vi "observacao.vi"() -> ()   [LabVIEW 2018, in "Shared_160.lvlib"] (continued)
                n1094 = case shown="True" w1420 {
                  selector: w1420 -> [_ w1423]
                  frame False {
                  }
                  frame True {
                    n1095 = Not(x=w1423) -> (.not. x?=w1422:bool)
                    n1096 = property on="Mensage Alarme" class="Str"("Visible"=FALSE) -> ()  [unwired: 2 in, 2 out]
                    n1097 = local write "Flag Alarm"(w1422) -> ()
                  }
                }
              }
            }
          }
          frame #13 {
            w1438 = u16 3 items=["Alarme", "Atencao", "Erro", "Ocupado", "Protecao", "Embreagem", "Tracking", "Var. Track", "Rápido", "Ligeiro", "Médio", "Lento", "Em movimento", ""] ("NomeStatus")
            w1439 = u16 3 items=["Alarme", "Atencao", "Erro", "Ocupado", "Protecao", "Embreagem", "Tracking", "Var. Track", "Rápido", "Ligeiro", "Médio", "Lento", "Em movimento", ""] ("NomeStatus")
            # "PROCESSO AQUISIÇÃO"
            n1098 = global read "Global_Telescopio.vi" "Correção Aquis"() -> (w1434:bool)
            n1099 = call "Bit Status AH.vi"("NomeStatus"=w1439) -> ("StatBit"=w1436:bool)
            n1100 = call "Bit Status DEC.vi"("NomeStatus"=w1438) -> ("StatBit"=w1437:bool)
            n1101 = Not Or(1:w1437, 2:w1436) -> (0:w1435:bool)
            n1102 = Compound Arithmetic op=AND(w1434, w1435) -> (w1440:bool)
            n1103 = case shown="True" w1440 {
              frame False {
              }
              frame True {
                # "Reseta Flag do movimento de\n offset do Sist de Aquisição"
                n1104 = global read "Global_Telescopio.vi" "CorrecaoMin"() -> (w1446:dbl)
                n1105 = global read "Global_Telescopio.vi" "aquis_asc"() -> (w1445:dbl)
                n1106 = global read "Global_Telescopio.vi" "aquis_dec"() -> (w1448:dbl)
                n1107 = Absolute Value(x=w1448) -> (abs(x)=w1444:dbl)
                n1108 = global read "Global_Telescopio.vi" "CorrecaoMin"() -> (w1449:dbl)
                n1109 = global write "Global_Telescopio.vi" "Correção Aquis"(FALSE ("Correção Aquis")) -> ()
                n1110 = Absolute Value(x=w1445) -> (abs(x)=w1443:dbl)
                n1111 = Greater?(x=w1444, y=w1449) -> (0:w1450:bool)
                n1112 = Greater?(x=w1443, y=w1446) -> (0:w1447:bool)
                n1113 = case shown="True" w1447 {
                  tunnel: w1445 -> [_ w1451]
                  frame False {
                  }
                  frame True {
                    w1453 = u16 1 items=["ZERO", "AH", "DEC", "TUBO", "CUP"] ("Controlador")
                    # "PROCESSO MOVE TELESCÓPIO"
                    n1114 = call "Conversao Ms to Hora texto.vi"("TRUE=HORA\nFALSE=GRAU"=TRUE ("TRUE=HORA\nFALSE=GRAU"), "PrecDEC"=w1451) -> ("Hora/Graus Texto Decimal"=w1456:string)
                    n1115 = call "Monta Comando.vi"("Set Point"=w1456, "Comando"="MOVER_REL", "Dispositivo"="EIXO" ("Comando"), "Controlador"=w1453) -> ()  [unwired: 1 in, 5 out]
                  }
                }
                n1116 = case shown="True" w1450 {
                  tunnel: w1448 -> [_ w1457]
                  frame False {
                  }
                  frame True {
                    w1459 = u16 2 items=["ZERO", "AH", "DEC", "TUBO", "CUP"] ("Controlador")
                    # "PROCESSO MOVE TELESCÓPIO"
                    n1117 = call "Conversao Ms to Hora texto.vi"("TRUE=HORA\nFALSE=GRAU"=FALSE ("TRUE=HORA\nFALSE=GRAU"), "PrecDEC"=w1457) -> ("Hora/Graus Texto Decimal"=w1462:string)
                    n1118 = call "Monta Comando.vi"("Set Point"=w1462, "Comando"="MOVER_REL", "Dispositivo"="EIXO" ("Comando"), "Controlador"=w1459) -> ()  [unwired: 1 in, 5 out]
                  }
                }
                n1119 = global write "Global_Telescopio.vi" "AQ Offset Mov"(TRUE ("AQ Offset Mov")) -> ()
              }
            }
          }
          frame #14 {
            w1475 = "\r\n"
            # "MUDANÇA 10/8/2010 \nIncluídos:\n- Nome do instrumento\n- RA do telescópio"
            # "OBS: O Arquivo é inicialmente apagado para \nEvitar que fique corrompido!"
            # "Escreve arquivo com Dados para o Uso da Página do PDA"
            n1120 = global read "Global_Telescopio.vi" "Lista Instrumentos"() -> (w1477:string[])
            n1121 = global read "Global_Telescopio.vi" "Sideral Time"() -> (w1467:dbl)
            n1122 = global read "Global_Telescopio.vi" "PosAH"() -> (w1468:dbl)
            n1123 = global read "Global_Telescopio.vi" "Instrum"() -> (w1476:u16)
            n1124 = local read "DOMO_ENC"() -> (w1489:string)
            n1125 = local read "CUP_STAT"() -> (w1485:string)
            n1126 = local read "AH_STAT"() -> (w1487:string)
            n1127 = local read "Sideral time"() -> (w1496:string)
            n1128 = local read "AH_ENC"() -> (w1491:string)
            n1129 = local read "UT"() -> (w1495:string)
            n1130 = Subtract(x=w1467, y=w1468) -> (x-y=w1472:dbl)
            n1131 = Add(x=6.283185307179586, y=w1472) -> (x+y=w1471:dbl)
            n1132 = Less Than 0?(x=w1472) -> (x < 0?=w1469:bool)
            n1133 = local read "TUBO_STAT"() -> (w1484:string)
            n1134 = call "Retira_tudo_depois_da_virgula.vi"("Entrada"=w1496) -> ("Saída"=w1493:string)
            n1135 = Format Date/Time String(time format string (%c)="%H:%M:%S") -> (date/time string=w1479:string)  [unwired: 2 in]
            n1136 = local read "FOCO_ENC"() -> (w1488:string)
            n1137 = local read "DEC_STAT"() -> (w1486:string)
            n1138 = local read "DEC_ENC"() -> (w1490:string)
            n1139 = Select(t=w1471, s=w1469, f=w1472) -> (s? t:f=w1473:dbl)
            n1140 = Index Array(array=w1477, index=w1476) -> (element=w1478:string)
            n1141 = Format Date/Time String(time format string (%c)="%d/%m/%Y") -> (date/time string=w1480:string)  [unwired: 2 in]
            n1142 = call "Retira_tudo_depois_da_virgula.vi"("Entrada"=w1495) -> ("Saída"=w1492:string)
            n1143 = call <vilib>:"Trim Whitespace.vi"("string"=w1493) -> ("trimmed string"=w1483:string)  [unwired: 1 in]
            n1144 = call "rad_hms.vi"("TRUE=HORA\nFALSE=GRAU"=TRUE, "Radiano"=w1473) -> ("Hora/Graus Texto Decimal"=w1466:string)  [unwired: 3 in]
            n1145 = String To Path(string="C:\\TCS\\ARQUIVOS\\DadosTCSPD.txt") -> (path=w1497:path)
            n1146 = Concatenate Strings(w1480, w1475, w1479, w1475, w1492, w1475, w1483, w1475, w1491, w1475, w1490, w1475, w1489, w1475, w1488, w1475, w1487, w1475, w1486, w1475, w1485, w1475, w1484, w1475, w1478, w1475, w1466, w1475) -> (w1499:string)
            n1147 = case shown="True" "Case Constant\n(See Context Help) 2" {
              tunnel: [w1508 w1511] -> w1498
              tunnel: w1497 -> [w1508 w1510]
              frame False {
              }
              frame True {
                n1148 = Delete(path (use dialog)=w1510) -> (deleted path=w1511:path, error out=→"error out":errorcluster)  [unwired: 4 in, 1 out]
              }
            }
            n1149 = call <vilib>:"Open_Create_Replace File.vi"("function (open:0)"=T8."open or create", "file path"=w1498) -> ("error out"=w1503:errorcluster, "refnum"=w1506:refnum<file>)  [unwired: 6 in, 2 out]
            n1150 = Set File Position(refnum=w1506, from (0:start)=enum16{"start", "end", "current"}."start" ("pos mode (0:2)"), error in=w1503) -> (refnum out=w1465:refnum<file>, error out=w1464:errorcluster)  [unwired: 1 in]
            n1151 = Write to Binary File(file (use dialog)=w1465, data=w1499, error in=w1464, 5:FALSE ("prepend array or string size? (T)")) -> (refnum out=w1505:refnum<file>, error out=w1504:errorcluster)  [unwired: 2 in, 1 out]
            n1152 = Close File(refnum=w1505, error in=w1504) -> (error out=w1507:errorcluster)  [unwired: 1 out]
            n1153 = call <vilib>:"Simple Error Handler.vi"("error in (no error)"=w1507) -> ()  [unwired: 4 in, 5 out]
          }
          frame #15 {
            # "Página do PDA"
            # "http://192.168.1.1:1080/pdaWeb/"
            # "TRATAMENTO DO PDA"
            n1154 = stacked-sequence {
              frame #0 {
                # "MUDANÇA  3/9/2010 \nIncluído case abaixo e código de seu estado TRUE para apagar eventuais comandos do PDA enviados antes do TCSPD rodar."
                n1155 = First Call?() -> (First Call?: T/F=w1512:bool)
                n1156 = case shown="True" w1512 {
                  frame False {
                    # "MUDANÇA  4/9/2010 \nSubstituída a VI \"New Read PPC\" pela \"Trata PDA\" a qual evita que o telescópio seja apontado para regiões proibidas (inclinação excessiva)."
                    # "lê e interpreta o arquivo ppc.txt"
                    n1157 = call "Trata PDA.vi"() -> ()  [unwired: 2 in]
                  }
                  frame True {
                    n1158 = call "Find ppctxt.vi"() -> ("Existe ppc.txt?"=w1514:bool, "ppc.txt Path"=w1513:path)  [unwired: 1 in]
                    n1159 = case shown="True" w1514 {
                      tunnel: w1513 -> [_ w1515]
                      frame False {
                      }
                      frame True {
                        # "limpa o arquivo ppc.txt"
                        n1160 = call "Wipe file.vi"("ppc path"=w1515) -> ()  [unwired: 2 out]
                      }
                    }
                  }
                }
              }
              frame #1 {
                n1161 = case shown="False" "Case Constant\n(See Context Help) 3" {
                  frame False {
                  }
                  frame True {
                    # "MUDANÇA:\nÉ necesário \nsubstituir as variáveis simuladas pelas do Sistema"
                    # "Simula os dados sendo alterados pela\nmovimentação do sistema"
                    n1162 = call "Data Table.vi"() -> ()  [unwired: 1 in]
                  }
                }
              }
              frame #2 {
                n1163 = case shown="True" "Case Constant\n(See Context Help) 4" {
                  frame False {
                  }
                  frame True {
                    # "Lê o arquivo padrão para o equip/o\nselecionado pelo PDA e grava o\narquivo ppcDisplay.htm adequado"
                    n1164 = call "Update Frame.vi"() -> ("Timeout"=w1518:u32)  [unwired: 2 in, 3 out]
                    n1165 = Wait Until Next ms Multiple(millisecond multiple=w1518) -> ()  [unwired: 1 out]
                  }
                }
              }
            }
          }
        }
        n1166 = global read "Global_Telescopio.vi" "Flag-Rotator"() -> (w99:bool)
        n1167 = case shown="True" w99 {
          frame False {
          }
          frame True {
            n1168 = local write "Setup, Pointing & Guiding"(T2."ROTATOR" ("Setup, Pointing & Guiding")) -> ()
          }
        }
      }
      frame #2 {
        n1169 = case shown="\"HANDSET\"" "Setup, Pointing & Guiding" {
          frame "POINTING", Default {
            n1170 = stacked-sequence {
              frame #0 {
                # "Clear Dados"
                n1171 = local read "ChkCalLocal"() -> (w1520:bool)
                n1172 = case shown="False" w1520 {
                  selector: w1520 -> [w1522 _]
                  frame False {
                    # "Para de Piscar/Blink\no botão"
                    n1173 = property on="ChkCalLocal" class="Bool (strict)"("Blinking"=w1522) -> ()  [unwired: 2 in, 2 out]
                  }
                  frame True {
                  }
                }
                n1174 = case shown="True" "BtPointObjClear" {
                  frame False {
                  }
                  frame True {
                    w1523 = ""
                    n1175 = local write "StrPointObjName"(w1523) -> ()
                    n1176 = local write "StrPointObjPMRA"(w1523) -> ()
                    n1177 = local write "StrPointObjPMDEC"(w1523) -> ()
                    n1178 = local write "StrPointObjRA"(w1523) -> ()
                    n1179 = local write "StrPointObjDEC"(w1523) -> ()
                    n1180 = local write "StrPointObjEpoch"(w1523) -> ()
                    n1181 = local write "StrPointTargetRA"(w1523) -> ()
                    n1182 = local write "StrPointTargetDEC"(w1523) -> ()
                  }
                }
              }
              frame #1 {
                # "20250910"
                # "20250910"
                # "A forma como os mostradores da janela TARGET são carregados está indefinida.\nVamos colocar um botão SET ao lado do botão CLEAR na janela OBJECT.\nQuando o botão SET for pressionado, os mostradores da janela TARGET\nseriam calculados a partir dos valores da janela OBJECT."
                n1183 = local read "StrPointObjRA"() -> (w1536:string)
                n1184 = local read "StrPointObjDEC"() -> (w1537:string)
                n1185 = local read "StrPointObjPMRA"() -> (w1527:string)
                n1186 = local read "StrPointObjPMDEC"() -> (w1526:string)
                n1187 = local read "Temp amb"() -> (w1542:string)
                n1188 = local read "pressão atm"() -> (w1541:string)
                n1189 = local read "hum local"() -> (w1540:string)
                n1190 = call "Check coord input.vi"("coordIn"=w1536, "RA=T, default: F=DEC"=TRUE) -> ("coordOut"=w1532:string, "valid"=w1531:bool)  [unwired: 8 in]
                n1191 = call "Check coord input.vi"("coordIn"=w1537, "RA=T, default: F=DEC"=FALSE) -> ("coordOut"=w1535:string, "valid"=w1534:bool)  [unwired: 8 in]
                n1192 = call "Arcsec to Rad_ String.vi"("VAR ARCSEC"=w1527) -> ("VAR RAD"=w1529:string, "valid"=w1524:bool)  [unwired: 5 in]
                n1193 = call "Arcsec to Rad_ String.vi"("VAR ARCSEC"=w1526) -> ("VAR RAD"=w1528:string, "valid"=w1525:bool)  [unwired: 5 in]
                n1194 = Compound Arithmetic op=AND("BtPointPrecess", w1531, w1534, w1524, w1525) -> (w1539:bool)
                n1195 = case shown="True" w1539 {
                  tunnel: w1532 -> [_ w1551]
                  tunnel: w1535 -> [_ w1550]
                  tunnel: w1542 -> [_ w1549]
                  tunnel: w1541 -> [_ w1548]
                  tunnel: w1540 -> [_ w1547]
                  tunnel: w1529 -> [_ w1546]
                  tunnel: w1528 -> [_ w1545]
                  tunnel: "BtPointPrecess" -> [w1543 _]
                  frame False {
                    n1196 = case shown="True" w1543 {
                      frame False {
                      }
                      frame True {
                        n1197 = One Button Dialog(message="Entrada inválida.\nInvalid data entry") -> ()  [unwired: 1 in, 1 out]
                      }
                    }
                  }
                  frame True {
                    n1198 = stacked-sequence {
                      tunnel: w1551 -> [w1587 _ _]
                      tunnel: w1550 -> [w1585 _ _]
                      tunnel: w1549 -> [w1595 _ _]
                      tunnel: w1548 -> [w1594 _ _]
                      tunnel: w1547 -> [w1593 _ _]
                      tunnel: w1546 -> [w1559 _ _]
                      tunnel: w1545 -> [w1558 _ _]
                      frame #0 {
                        # "PROCESSO PRECESSÃO"
                        # "MUDANÇA:\nVI Botao SET trocada por Botao Precess, eliminando entrada do Frame de coord. (Mean, Topo, Geo)"
                        n1199 = local read "ChkPointPrecessed"() -> (w1567:bool)
                        n1200 = call "Comma_to_Point.vi"("Lat_A"=w1585) -> ("Saída"=w1581:string)
                        n1201 = call "Comma_to_Point.vi"("Lat_A"=w1587) -> ("Saída"=w1583:string)
                        n1202 = call "hms_rad.vi"("True = hora"=FALSE, "Texto Graus"=w1581) -> ("radianos"=w1554:dbl)  [unwired: 3 in]
                        n1203 = call "hms_rad.vi"("True = hora"=TRUE, "Texto Graus"=w1583) -> ("radianos"=w1557:dbl)  [unwired: 3 in]
                        n1204 = call "rad_hms.vi"("TRUE=HORA\nFALSE=GRAU"=TRUE ("TRUE=HORA\nFALSE=GRAU"), "Radiano"=w1557) -> ("Hora/Graus Texto Decimal"=w1555:string)  [unwired: 3 in]
                        n1205 = call "rad_hms.vi"("TRUE=HORA\nFALSE=GRAU"=FALSE ("TRUE=HORA\nFALSE=GRAU"), "Radiano"=w1554) -> ("Hora/Graus Texto Decimal"=w1553:string)  [unwired: 3 in]
                        n1206 = call "Comma_to_Point.vi"("Lat_A"=w1594) -> ("Saída"=w1565:string)
                        n1207 = call "Comma_to_Point.vi"("Lat_A"=w1593) -> ("Saída"=w1564:string)
                        n1208 = call "Comma_to_Point.vi"("Lat_A"=w1595) -> ("Saída"=w1566:string)
                        n1209 = global write "Global_Telescopio.vi" "pubRaAcquis"(w1555) -> ()
                        n1210 = global write "Global_Telescopio.vi" "pubDecAcquis"(w1553) -> ()
                        n1211 = Number To Fractional String(use system decimal point (T)=FALSE, number=w1554, precision (6)=i16 9) -> (F-format string=w1570:string)  [unwired: 1 in]
                        n1212 = Number To Fractional String(use system decimal point (T)=FALSE, number=w1557, precision (6)=i16 9) -> (F-format string=w1571:string)  [unwired: 1 in]
                        n1213 = call "Botão Precess.vi"("AR"=w1571, "Precessed Coord."=w1567, "Dec"=w1570, "Temp local amb(K)"=w1566, "Pressao atm local (mB)"=w1565, "Hum rel local"=w1564, "Var RA"=w1559, "Var DEC"=w1558) -> ("RA"=w1597:dbl, "DEC"=w1560:dbl, "Hora Sideral (rad)"=w1596:dbl, "Dist. Zenital (rad)"=w1569:dbl, "Observed HA (radians)"=→"HA obs":dbl, "Massa de Ar"=w1568:dbl)  [unwired: 2 in]
                        "RA obs" <- w1597
                        "DEC obs" <- w1560
                        n1214 = local write "Zenital angle"(w1569) -> ()
                        n1215 = call "rad_hms.vi"("TRUE=HORA\nFALSE=GRAU"=FALSE ("TRUE=HORA\nFALSE=GRAU"), "Radiano"=w1560) -> ("Hora/Graus Texto Decimal"=w1577:string)  [unwired: 3 in]
                        n1216 = call "rad-graus.vi"("Radiano"=w1569) -> ("Graus"=w1592:dbl)
                        n1217 = Number To Fractional String(number=w1568, precision (6)=i16 3) -> (F-format string=→"Air Mass":string)  [unwired: 2 in]
                        n1218 = Number To Fractional String(number=w1592, precision (6)=i16 1) -> (F-format string=→"Zenital Angle":string)  [unwired: 2 in]
                        n1219 = call "rad_hms.vi"("TRUE=HORA\nFALSE=GRAU"=TRUE ("TRUE=HORA"), "Radiano"=w1597) -> ("Hora/Graus Texto Decimal"=w1579:string)  [unwired: 3 in]
                        n1220 = local write "StrPointTargetDEC"(w1577) -> ()
                        n1221 = local write "StrPointTargetRA"(w1579) -> ()
                        n1222 = disable-structure shown="Disabled" {
                          disable-tunnel: [w1601 _] -> _
                          disable-tunnel: w1597 -> [w1600 _]
                          disable-tunnel: w1596 -> [w1599 _]
                          disable-tunnel: w1560 -> [w1598 _]
                          frame Disabled {
                            n1223 = call "Hora_Limite.vi"("Asc Reta RA rad"=w1600, "Sideral Time rad"=w1599, "Declinação rad"=w1598) -> ("TO Tempo de Observação Horas"=w1601:dbl)  [unwired: 2 in]
                          }
                          frame Enabled {
                          }
                        }
                        n1224 = call "Novo_tempo_obs_inicial.vi"("TS"=w1596, "RA"=w1597, "DEC"=w1560) -> ("TO rad"=w1561:dbl)  [unwired: 7 in, 1 out]
                        n1225 = case shown="True" "TRUE=HORA\nFALSE=GRAU" {
                          frame False {
                          }
                          frame True {
                            # "Sincroniza hora do\nPC com GPS"
                            n1226 = call "About_Time.vi"() -> ()  [unwired: 1 in]
                          }
                        }
                        n1227 = call "rad_hms.vi"("TRUE=HORA\nFALSE=GRAU"=TRUE ("TRUE=HORA\nFALSE=GRAU"), "Radiano"=w1561) -> ("Hora/Graus Texto Decimal"=→"Tempo Obs":string)  [unwired: 3 in]
                      }
                      frame #1 {
                        # "Testa o ângulo zenital menor que 70º o led \"Working Area\" \naceso na cor verde se o ângulozenital menor que 70º e \nvermelho em caso cont rário."
                        n1228 = global read "Global_Telescopio.vi" "Piscar working area"() -> (w1608:bool)
                        n1229 = global read "Global_Telescopio.vi" "working area = VERDE"() -> (w1607:bool)
                        n1230 = global read "Global_Telescopio.vi" "ativar botão GO"() -> (w1605:bool)
                        n1231 = case shown="True" w1607 {
                          frame False {
                            # "False=Vermelho"
                            n1232 = local write "LedPointWorkArea"(FALSE ("LedPointWorkArea")) -> ()
                          }
                          frame True {
                            # "True=Verde"
                            "LedPointWorkArea" <- TRUE ("LedPointWorkArea")
                          }
                        }
                        n1233 = global write "Global_Telescopio.vi" "Botão GO = STOP"(FALSE ("Botão GO = STOP")) -> ()
                        n1234 = case shown="True" w1605 {
                          selector: w1605 -> [_ w1609]
                          frame False {
                          }
                          frame True {
                            n1235 = property on="BtTargetPoint" class="Bool"("Visible"=w1609) -> ()  [unwired: 2 in, 2 out]
                          }
                        }
                        n1236 = global write "Global_Telescopio.vi" "Piscar working area"(w1608) -> ()
                        n1237 = global read "Global_Telescopio.vi" "desativar botão GO"() -> (w1606:bool)
                        n1238 = case shown="True" w1606 {
                          selector: w1606 -> [_ w1611]
                          frame False {
                          }
                          frame True {
                            n1239 = Not(x=w1611) -> (.not. x?=w1610:bool)
                            n1240 = property on="BtTargetPoint" class="Bool"("Visible"=w1610) -> ()  [unwired: 2 in, 2 out]
                          }
                        }
                        n1241 = property on="LedPointWorkArea" class="Bool (strict)"("Visible"=TRUE ("Botão GO = STOP")) -> ()  [unwired: 2 in, 2 out]
                        n1242 = property on="LedPointing" class="Bool (strict)"("Visible"=FALSE) -> ()  [unwired: 2 in, 2 out]
                      }
                      frame #2 {
                        n1243 = global read "Global_Telescopio.vi" "CalDEC Local"() -> (w1619:dbl)
                        n1244 = global read "Global_Telescopio.vi" "CalAH Local"() -> (w1620:dbl)
                        n1245 = local read "ChkCalLocal"() -> (w1614:bool)
                        n1246 = Not Equal To 0?(x=w1620) -> (x != 0?=w1617:bool)
                        n1247 = Not Equal To 0?(x=w1619) -> (x != 0?=w1618:bool)
                        n1248 = Or(x=w1617, y=w1618) -> (x .or. y?=w1615:bool)
                        n1249 = And(x=w1614, y=w1615) -> (x .and. y?=w1616:bool)
                        n1250 = case shown="True" w1616 {
                          frame False {
                          }
                          frame True {
                            n1251 = local read "HA obs"() -> (w1640:dbl)
                            n1252 = local read "DEC obs"() -> (w1634:dbl)
                            n1253 = global read "Global_Telescopio.vi" "AH Zero Local"() -> (w1638:dbl)
                            n1254 = global read "Global_Telescopio.vi" "DEC Zero Local"() -> (w1633:dbl)
                            n1255 = global read "Global_Telescopio.vi" "Raio Máximo"() -> (w1622:dbl)
                            n1256 = Cosine(x=w1634) -> (cos(x)=w1639:dbl)
                            n1257 = Cosine(x=w1633) -> (cos(x)=w1637:dbl)
                            n1258 = Multiply(x=w1640, y=w1639) -> (x*y=w1636:dbl)
                            n1259 = Multiply(x=w1638, y=w1637) -> (x*y=w1635:dbl)
                            n1260 = Subtract(x=w1634, y=w1633) -> (x-y=w1629:dbl)
                            n1261 = Multiply(x=w1629, y=w1629) -> (x*y=w1632:dbl)
                            n1262 = Subtract(x=w1636, y=w1635) -> (x-y=w1628:dbl)
                            n1263 = Multiply(x=w1628, y=w1628) -> (x*y=w1630:dbl)
                            n1264 = Add(x=w1630, y=w1632) -> (x+y=w1631:dbl)
                            n1265 = Square Root(x=w1631) -> (sqrt(x)=w1627:dbl)
                            n1266 = Multiply(x=w1627, y=180.0) -> (x*y=w1625:dbl)
                            n1267 = Divide(x=w1625, y=3.141592653589793) -> (x/y=w1623:dbl)
                            n1268 = Greater?(x=w1623, y=w1622) -> (0:w1621:bool)
                            n1269 = property on="ChkCalLocal" class="Bool (strict)"("Blinking"=w1621) -> ()  [unwired: 2 in, 2 out]
                          }
                        }
                      }
                    }
                  }
                }
              }
              frame #2 {
                # "20250910"
                # "Clicando-se essa Tecla\nInicia-se o Apontamento"
                n1270 = local read "StrPointObjRA"() -> (w1655:string)
                n1271 = local read "StrPointObjDEC"() -> (w1652:string)
                n1272 = local read "StrPointObjPMRA"() -> (w1642:string)
                n1273 = local read "StrPointObjPMDEC"() -> (w1643:string)
                n1274 = local read "Temp amb"() -> (w1658:string)
                n1275 = local read "pressão atm"() -> (w1657:string)
                n1276 = local read "hum local"() -> (w1663:string)
                n1277 = control-ref of="BtTargetPoint"() -> (w1660:refnum<vi>)
                n1278 = property class="Bool"(reference=w1660) -> ("Boolean Text.Text"=w1661:string)  [unwired: 1 in, 2 out]
                n1279 = call "Check coord input.vi"("coordIn"=w1655, "RA=T, default: F=DEC"=TRUE) -> ("coordOut"=w1653:string, "valid"=w1649:bool)  [unwired: 8 in]
                n1280 = call "Check coord input.vi"("coordIn"=w1652, "RA=T, default: F=DEC"=FALSE) -> ("coordOut"=w1651:string, "valid"=w1648:bool)  [unwired: 8 in]
                n1281 = call "Arcsec to Rad_ String.vi"("VAR ARCSEC"=w1642) -> ("VAR RAD"=w1644:string, "valid"=w1646:bool)  [unwired: 5 in]
                n1282 = call "Arcsec to Rad_ String.vi"("VAR ARCSEC"=w1643) -> ("VAR RAD"=w1645:string, "valid"=w1647:bool)  [unwired: 5 in]
                n1283 = Equal?(x=w1661, y="POINT") -> (x = y?=w1659:bool)
                n1284 = Compound Arithmetic op=AND("BtTargetPoint", w1649, w1648, w1646, w1647) -> (w1656:bool)
                n1285 = case shown="True" w1656 {
                  tunnel: w1653 -> [_ w1670]
                  tunnel: w1651 -> [_ w1674]
                  tunnel: w1658 -> [_ w1671]
                  tunnel: w1657 -> [_ w1672]
                  tunnel: w1663 -> [_ w1673]
                  tunnel: w1659 -> [_ w1668]
                  tunnel: w1645 -> [_ w1667]
                  tunnel: w1644 -> [_ w1666]
                  tunnel: "BtTargetPoint" -> [w1664 _]
                  frame False {
                    n1286 = case shown="True" w1664 {
                      frame False {
                      }
                      frame True {
                        n1287 = One Button Dialog(message="Entrada inválida.\nInvalid data entry") -> ()  [unwired: 1 in, 1 out]
                      }
                    }
                  }
                  frame True {
                    n1288 = case shown="True" w1668 {
                      selector: w1668 -> [w1676 _]
                      tunnel: w1674 -> [_ w1700]
                      tunnel: w1673 -> [_ w1686]
                      tunnel: w1672 -> [_ w1685]
                      tunnel: w1671 -> [_ w1684]
                      tunnel: w1670 -> [_ w1699]
                      tunnel: w1667 -> [_ w1679]
                      tunnel: w1666 -> [_ w1680]
                      frame False {
                        w1677 = 0 ("estado")
                        # "Zera Máquina de Estado\nPelo Botão STOP"
                        n1289 = Not(x=w1676) -> (.not. x?=w1678:bool)
                        n1290 = local write "LedPointing"(w1676) -> ()
                        n1291 = global write "Global_Telescopio.vi" "Botão GO = STOP"(w1678) -> ()
                        n1292 = call "Stop.vi"() -> ()  [unwired: 1 in, 1 out]
                        n1293 = local write "statDEC"(w1677) -> ()
                        n1294 = local write "statAH"(w1677) -> ()
                        n1295 = local write "statCUP"(w1677) -> ()
                        "Flag Stop" <- TRUE ("Flag Stop")
                      }
                      frame True {
                        w1681 = ""
                        w1698 = FALSE ("use system decimal point (T)")
                        n1296 = call "Comma_to_Point.vi"("Lat_A"=w1699) -> ("Saída"=w1694:string)
                        n1297 = call "Comma_to_Point.vi"("Lat_A"=w1700) -> ("Saída"=w1695:string)
                        n1298 = call "hms_rad.vi"("True = hora"=TRUE, "Texto Graus"=w1694) -> ("radianos"=w1703:dbl)  [unwired: 3 in]
                        n1299 = call "hms_rad.vi"("True = hora"=FALSE, "Texto Graus"=w1695) -> ("radianos"=w1701:dbl)  [unwired: 3 in]
                        n1300 = local write "NAME"(w1681) -> ()
                        n1301 = local write "RA"(w1681) -> ()
                        n1302 = local write "DEC"(w1681) -> ()
                        n1303 = Number To Fractional String(use system decimal point (T)=w1698, number=w1703, precision (6)=i16 9) -> (F-format string=w1683:string)  [unwired: 1 in]
                        n1304 = Number To Fractional String(use system decimal point (T)=w1698, number=w1701, precision (6)=i16 9) -> (F-format string=w1682:string)  [unwired: 1 in]
                        n1305 = call "PrecessaoCorrigida.vi"("Coordenada do dia"="ChkPointPrecessed", "HabCorrModelo"="ChkModel", "UseLocalZero"="ChkCalLocal", "UseGlobalZero"="ChkCalGlobal", "RA"=w1683, "DEC"=w1682, "MovProprioRA"=w1680, "MovProprioDEC"=w1679, "Temp amb (K)"=w1684, "Press atm (mB)"=w1685, "Humid relat"=w1686) -> ("Estado"=w1689:i32, "RA"=w1688:dbl, "DEC"=w1687:dbl)  [unwired: 2 out]
                        n1306 = Equal To 0?(x=w1689) -> (x = 0?=w1696:bool)
                        n1307 = case shown="False" w1696 {
                          selector: w1696 -> [w1719 _]
                          tunnel: "ChkCalLocal" -> [w1731 _]
                          tunnel: "ChkCalGlobal" -> [w1730 _]
                          tunnel: w1682 -> [w1729 _]
                          tunnel: w1683 -> [w1728 _]
                          tunnel: w1679 -> [w1725 _]
                          tunnel: w1680 -> [w1724 _]
                          tunnel: w1689 -> [w1706 _]
                          tunnel: w1688 -> [w1727 _]
                          tunnel: w1687 -> [w1726 _]
                          tunnel: "ChkPointPrecessed" -> [w1722 _]
                          frame False {
                            w1709 = FALSE ("Coude")
                            w1710 = FALSE ("WeakSel")
                            w1711 = T5."Enabled" ("Disabled")
                            w1712 = TRUE ("MOUNT")
                            w1723 = 0 ("M_AH")
                            w1720 = TRUE
                            # "ABAS DE CONTROLE"
                            # "MUDANÇA:\nIncluído CASE"
                            # "Seta máquinas de\nestado aba ÚTILS"
                            n1308 = global write "Global_Telescopio.vi" "CoordDia"(w1722) -> ()
                            n1309 = global write "Global_Telescopio.vi" "CalGlobal"(w1730) -> ()
                            n1310 = global write "Global_Telescopio.vi" "CalLocal"(w1731) -> ()
                            n1311 = call "Envia LOG.vi"() -> ()  [unwired: 8 in, 2 out]
                            n1312 = global write "Global_Telescopio.vi" "TargetRA"(w1727) -> ()
                            n1313 = global write "Global_Telescopio.vi" "TargetDEC"(w1726) -> ()
                            n1314 = local write "statAH"(w1706) -> ()
                            n1315 = property on="LedPointWorkArea" class="Bool (strict)"("Visible"=FALSE ("Botão GO = STOP")) -> ()  [unwired: 2 in, 2 out]
                            n1316 = local write "statDEC"(w1706) -> ()
                            n1317 = global write "Global_Telescopio.vi" "ObjCentrado"(w1719) -> ()
                            n1318 = local write "RA on Target"(w1719) -> ()
                            n1319 = local write "DEC on Target"(w1719) -> ()
                            n1320 = local write "Dome on Target"(w1719) -> ()
                            n1321 = local read "ChkDomeEnable"() -> (w1718:bool)
                            n1322 = local write "M_AH"(w1723) -> ()
                            n1323 = local write "M_DEC"(w1723) -> ()
                            n1324 = local write "M_CUP"(w1723) -> ()
                            n1325 = case shown="True" w1718 {
                              selector: w1718 -> [w1752 _]
                              tunnel: w1706 -> [_ w1754]
                              tunnel: [0 ("Estado") w1754] -> w1717
                              tunnel: [u8 2 ("Disabled") u8 0 ("Disabled")] -> w1716
                              frame False {
                                n1326 = local write "DOME"(w1752) -> ()
                              }
                              frame True {
                              }
                            }
                            n1327 = Tick Count (ms)() -> (millisecond timer value=w1714:u32)
                            n1328 = Add(x=w1714, y=u32 120000) -> (x+y=w1715:u32)
                            n1329 = local write "Tick Cupula"(w1715) -> ()
                            n1330 = local write "MOUNT"(w1712) -> ()
                            n1331 = local write "GUIDER"(w1712) -> ()
                            n1332 = property on="LedPointing" class="Bool (strict)"("Visible"=w1720) -> ()  [unwired: 2 in, 2 out]
                            n1333 = local write "statCUP"(w1717) -> ()
                            n1334 = property on="DOME" class="Bool (strict)"("Disabled"=w1716) -> ()  [unwired: 2 in, 2 out]
                            n1335 = stacked-sequence {
                              frame #0 {
                                n1336 = local read "StrPointObjName"() -> (w1732:string)
                                n1337 = local read "StrPointObjRA"() -> (w1733:string)
                                n1338 = local read "StrPointObjDEC"() -> (w1734:string)
                                n1339 = global write "Global_Telescopio.vi" "NAME OBJETO AUX"(w1732) -> ()
                                n1340 = global write "Global_Telescopio.vi" "RA AUX"(w1733) -> ()
                                n1341 = global write "Global_Telescopio.vi" "DEC AUX"(w1734) -> ()
                              }
                              frame #1 {
                                w1736 = u16 4 items=["ZERO", "AH", "DEC", "TUBO", "CUP"] ("Controlador")
                                n1342 = call "Monta Comando.vi"("Comando"="DESLIGAR", "Dispositivo"="FLAT_WEAK", "Controlador"=w1736) -> ()  [unwired: 2 in, 5 out]
                              }
                              frame #2 {
                                w1739 = u16 4 items=["ZERO", "AH", "DEC", "TUBO", "CUP"] ("Controlador")
                                n1343 = call "Monta Comando.vi"("Comando"="DESLIGAR", "Dispositivo"="FLAT_LO", "Controlador"=w1739) -> ()  [unwired: 2 in, 5 out]
                              }
                              frame #3 {
                                w1742 = u16 4 items=["ZERO", "AH", "DEC", "TUBO", "CUP"] ("Controlador")
                                n1344 = call "Monta Comando.vi"("Comando"="DESLIGAR", "Dispositivo"="FLAT_HI", "Controlador"=w1742) -> ()  [unwired: 2 in, 5 out]
                              }
                              frame #4 {
                                w1744 = u16 4 items=["ZERO", "AH", "DEC", "TUBO", "CUP"] ("Controlador")
                                n1345 = call "Monta Comando.vi"("Comando"="DESLIGAR", "Dispositivo"="FLAT_COUDE", "Controlador"=w1744) -> ()  [unwired: 2 in, 5 out]
                              }
                              frame #5 {
                                w1747 = u16 4 items=["ZERO", "AH", "DEC", "TUBO", "CUP"] ("Controlador")
                                n1346 = call "Monta Comando.vi"("Comando"="LIGAR", "Dispositivo"="LAMP_CAM", "Controlador"=w1747) -> ()  [unwired: 2 in, 5 out]
                              }
                              frame #6 {
                                n1347 = call "Log_Apontamento.vi"() -> ()  [unwired: 12 in]
                              }
                            }
                            n1348 = local write "DOME"(FALSE ("WeakSel")) -> ()
                            n1349 = local write "WeakSel"(w1710) -> ()
                            n1350 = local write "MediumSel"(w1710) -> ()
                            n1351 = local write "StrongSel"(w1710) -> ()
                            n1352 = local write "CoudeSel"(w1710) -> ()
                            n1353 = local write "Coude"(w1709) -> ()
                            n1354 = local write "Weak"(w1709) -> ()
                            n1355 = local write "Medium"(w1709) -> ()
                            n1356 = local write "Strong"(w1709) -> ()
                            n1357 = property on="Medium" class="Bool (strict)"("Disabled"=w1711) -> ()  [unwired: 2 in, 2 out]
                            n1358 = property on="Strong" class="Bool (strict)"("Disabled"=w1711) -> ()  [unwired: 2 in, 2 out]
                            n1359 = property on="Coude" class="Bool (strict)"("DisabledEnum"=w1711) -> ()  [unwired: 2 in, 2 out]
                            n1360 = property on="Weak" class="Bool (strict)"("Disabled"=w1711) -> ()  [unwired: 2 in, 2 out]
                            "MeanDEC" <- w1729
                            "MeanRA" <- w1728
                            "LedPointing" <- w1720
                            "PM_DEC" <- w1725
                            "PM_RA" <- w1724
                            "Apontou" <- TRUE ("WeakSel")
                          }
                          frame True {
                          }
                        }
                      }
                    }
                    n1361 = property on="Delete Calagem" class="Bool"("Disabled"=u8 0) -> ()  [unwired: 2 in, 2 out]
                  }
                }
              }
              frame #3 {
                # "e o led \"Working Area\" aceso na cor verde se o ângulo\nzenital menor que 70º e vermelho em caso cont rário.\nO botão GO ao ser clicado dispara o apontamento virtual do telescópio. Caso esse\nbotão seja pressionado enquanto o led \"Working Area\" est iver vermelho, este deve\npiscar 3 vezes e nada mais é executado. Caso cont rário, o nome do botão GO passa\npara CANCEL e o led \"Mount in Posit ion\" da janela STATUS INFORMATION deve ser\ndesligado, o que provocará a simulação do apontamento do telescópio (cf. item 4.3) .\nOs valores dos comandos \"Epoch\" , \"RA Proper Mot ion\" e \"DEC Proper Mot ion\" desse\nquadro devem ser ignorados na simulação."
                # "Habilita Cancela"
                # "Habilita Apontamento"
                n1362 = case shown="True" "Case Constant\n(See Context Help) 5" {
                  frame False {
                  }
                  frame True {
                    w1760 = TRUE ("Go aux")
                    w1761 = ""
                    n1363 = local write "DEC"(w1761) -> ()
                    n1364 = local write "RA"(w1761) -> ()
                    n1365 = local write "NAME"(w1761) -> ()
                    n1366 = control-ref of="BtTargetPoint"() -> (w1762:refnum<vi>)
                    n1367 = local write "LED MOUNT"(w1760) -> ()
                    n1368 = local write "MOUNT"(w1760) -> ()
                    n1369 = property class="Bool"(reference=w1762, "Boolean Text.Text"="STOP") -> ()  [unwired: 1 in, 2 out]
                  }
                }
                n1370 = case shown="True" "Case Constant\n(See Context Help) 6" {
                  frame False {
                  }
                  frame True {
                    w1757 = FALSE ("Go aux")
                    # "Seta nome para GO"
                    n1371 = local write "LED MOUNT"(w1757) -> ()
                    n1372 = local write "MOUNT"(w1757) -> ()
                    n1373 = control-ref of="BtTargetPoint"() -> (w1758:refnum<vi>)
                    n1374 = property class="Bool"(reference=w1758, "Boolean Text.Text"="POINT") -> ()  [unwired: 1 in, 2 out]
                  }
                }
              }
              frame #4 {
                # "Detecta Edição"
                # "os valores de RA e DEC devem assumir os valores da janela OBJECT da aba POINTING ao TÉRMINO do apontamento. Durante o apontamento devem ficar apagados. Como o campo MAG daquela janela não tem um valor correspondente na janela OBJECT, o campo MAG deve ficar em branco. Apenas quando as coordenadas da janela OBJECT da aba POINTING forem preenchidos a partir do botão SET COORD da aba LIST é que o campo MAG da janela TARGET assume o valor da coluna MAG da aba LIST. Colocar um flag interno (invisível para o usuário) para definir se o campo MAG deve ou não ser preenchido com o valor da aba LIST. Quando o botão SET COORD. fosse pressionado esse flag assumiria o valor verdadeiro e caso ocorresse edição dos valores da janela \nOBJECT da aba POINTING, esse flag assumiria o valor falso e o campo MAG da janela TARGET (entre os controles das abas e as imagens) ficaria vazio durante e após o apontamento"
                n1375 = local read "StrPointObjPMRA"() -> (w1777:string)
                n1376 = local read "StrPointObjPMDEC"() -> (w1776:string)
                n1377 = local read "StrPointObjName"() -> (w1784:string)
                n1378 = local read "AUX EDITA Name"() -> (w1783:string)
                n1379 = local read "StrPointObjEpoch"() -> (w1778:string)
                n1380 = local read "AUX EDITA EPOCH"() -> (w1773:string)
                n1381 = local read "AUX EDITA PMRA"() -> (w1774:string)
                n1382 = local read "AUX EDITA PMDEC"() -> (w1775:string)
                n1383 = local read "StrPointObjRA"() -> (w1782:string)
                n1384 = local read "StrPointObjDEC"() -> (w1780:string)
                n1385 = local read "AUX EDITA RA"() -> (w1781:string)
                n1386 = local read "AUX EDITA DEC"() -> (w1779:string)
                n1387 = Not Equal?(x=w1777, y=w1774) -> (x != y?=w1768:bool)
                n1388 = Not Equal?(x=w1784, y=w1783) -> (x != y?=w1772:bool)
                n1389 = Not Equal?(x=w1778, y=w1773) -> (x != y?=w1769:bool)
                n1390 = Not Equal?(x=w1776, y=w1775) -> (x != y?=w1767:bool)
                n1391 = Not Equal?(x=w1782, y=w1781) -> (x != y?=w1771:bool)
                n1392 = Not Equal?(x=w1780, y=w1779) -> (x != y?=w1770:bool)
                n1393 = Compound Arithmetic op=OR(w1772, w1771, w1770, w1769, w1768, w1767) -> (w1764:bool)
                n1394 = local read "FLAG SET COORD"() -> (w1765:bool)
                n1395 = And(x=w1764, y=w1765) -> (x .and. y?=w1766:bool)
                n1396 = case shown="True" w1766 {
                  frame False {
                  }
                  frame True {
                    # "Se houver edição o flag é resetado"
                    n1397 = local write "MAG"("") -> ()
                    "FLAG SET COORD" <- FALSE ("FLAG SET ACOORD")
                  }
                }
              }
            }
          }
          frame "HANDSET" {
            # "PROCESSO DISPLAY DESLOCAMENTO"
            n1398 = local read "AtualDEC"() -> (w1800:dbl)
            n1399 = global read "Global_Telescopio.vi" "Sideral Time"() -> (w1793:dbl)
            n1400 = global read "Global_Telescopio.vi" "PosAH"() -> (w1791:dbl)
            n1401 = Multiply(x="Velocity (arcsec/sec)", y=100.0) -> (x*y=w1808:dbl)
            n1402 = Cosine(x=w1800) -> (cos(x)=w1799:dbl)
            n1403 = Subtract(x=w1793, y=w1791) -> (x-y=w1792:dbl)
            n1404 = Absolute Value(x=w1799) -> (abs(x)=w1796:dbl)
            n1405 = Add(x=1e-10, y=w1796) -> (x+y=w1798:dbl)
            n1406 = local read "LatchDeslocRA"() -> (w1804:dbl)
            n1407 = local read "LatchDeslocDEC"() -> (w1803:dbl)
            n1408 = global read "Global_Telescopio.vi" "PosDEC"() -> (w1794:dbl)
            n1409 = event shown="[1] \"Left HS\": Value Change" {
              selector: _ -> [_ _ _ _ _ _ _ _ _ _ _]
              dyn-events: _ -> [_ _ _ _ _ _ _ _ _ _ _]
              timeout: 10 -> [_ _ _ _ _ _ _ _ _ _ _]
              tunnel: w1808 -> [_ w1821 w1829 w1837 _ _ _ _ _ _ w1940]
              tunnel: "Global" -> [_ _ _ _ _ _ _ _ w1882 w1902 _]
              tunnel: w1792 -> [_ _ _ _ w1840 _ _ _ _ w1900 _]
              tunnel: w1794 -> [_ _ _ _ _ w1841 _ _ _ w1901 _]
              tunnel: w1798 -> [_ _ _ _ _ _ w1842 w1860 _ _ _]
              event Timeout {
                n1410 = event-data() -> ()  [unwired: 1 in, 2 out]
              }
              event "Left HS": Value Change {
                w1818 = u8 0 ("Disabled")
                n1411 = event-data() -> ("NewVal"=w1817:bool)  [unwired: 1 in, 5 out]
                "MOV_IDX_AH" <- w1817
                n1412 = call "Tx handeset.vi"("CMD On"="left" ("Comando"), "CMD Off"="stoph" ("Comando"), "Estado do Botão"=w1817, "Velocity (arcsec/sec)"=w1821) -> ()  [unwired: 12 in]
                n1413 = Select(t=u8 2 ("Disabled"), s=FALSE, f=w1818) -> (s? t:f=w1819:u8)
                n1414 = property on="Delete Calagem" class="Bool"("Disabled"=w1818) -> ()  [unwired: 2 in, 2 out]
                n1415 = property on="Right HS" class="Bool (strict)"("Disabled"=w1819) -> ()  [unwired: 2 in, 2 out]
              }
              event "Down HS": Value Change {
                w1825 = u8 0 ("Disabled")
                n1416 = event-data() -> ("NewVal"=w1828:bool)  [unwired: 1 in, 5 out]
                "MOV_IDX_DEC" <- w1828
                n1417 = call "Tx handeset.vi"("CMD On"="down" ("Comando"), "CMD Off"="stopv" ("Comando"), "Estado do Botão"=w1828, "Velocity (arcsec/sec)"=w1829) -> ()  [unwired: 12 in]
                n1418 = Select(t=u8 2 ("Disabled"), s=FALSE, f=w1825) -> (s? t:f=w1826:u8)
                n1419 = property on="Delete Calagem" class="Bool"("Disabled"=w1825) -> ()  [unwired: 2 in, 2 out]
                n1420 = property on="Up HS" class="Bool (strict)"("Disabled"=w1826) -> ()  [unwired: 2 in, 2 out]
              }
              event "Right HS": Value Change {
                w1834 = u8 0 ("Disabled")
                n1421 = event-data() -> ("NewVal"=w1833:bool)  [unwired: 1 in, 5 out]
                n1422 = call "Tx handeset.vi"("CMD On"="right" ("Comando"), "CMD Off"="stoph" ("Comando"), "Estado do Botão"=w1833, "Velocity (arcsec/sec)"=w1837) -> ()  [unwired: 12 in]
                n1423 = local write "MOV_IDX_AH"(w1833) -> ()
                n1424 = Select(t=u8 2 ("Disabled"), s=FALSE, f=w1834) -> (s? t:f=w1835:u8)
                n1425 = property on="Delete Calagem" class="Bool"("Disabled"=w1834) -> ()  [unwired: 2 in, 2 out]
                n1426 = property on="Left HS" class="Bool (strict)"("Disabled"=w1835) -> ()  [unwired: 2 in, 2 out]
              }
              event "ClearDeslocRA": Value Change {
                n1427 = event-data() -> ()  [unwired: 1 in, 6 out]
                "LatchDeslocRA" <- w1840
              }
              event "ClearDeslocDEC": Value Change {
                n1428 = event-data() -> ()  [unwired: 1 in, 6 out]
                "LatchDeslocDEC" <- w1841
              }
              event "BtPrecCentrar": Value Change {
                # "PROCESSO OFFSET"
                n1429 = event-data() -> ()  [unwired: 1 in, 6 out]
                n1430 = stacked-sequence {
                  tunnel: w1842 -> [_ w1851]
                  frame #0 {
                    n1431 = local read "Offset DEC"() -> (w1843:dbl)
                    n1432 = Negate(x=w1843) -> (-x=w1844:dbl)
                    n1433 = Equal To 0?(x=w1843) -> (x = 0?=w1845:bool)
                    n1434 = case shown="False" w1845 {
                      tunnel: w1844 -> [w1846 _]
                      frame False {
                        n1435 = call "Conversao Ms to Hora texto.vi"("TRUE=HORA\nFALSE=GRAU"=FALSE ("TRUE=HORA\nFALSE=GRAU"), "PrecDEC"=w1846) -> ("Hora/Graus Texto Decimal"=w1848:string)
                        n1436 = call "Tx handeset.vi"("CMD On"="goDEC", "Set Point"=w1848, "Estado do Botão"=TRUE ("TRUE=HORA\nFALSE=GRAU")) -> ()  [unwired: 13 in]
                      }
                      frame True {
                      }
                    }
                  }
                  frame #1 {
                    # "PROCESSO MOVE TELESCÓPIO"
                    n1437 = local read "Offset RA"() -> (w1852:dbl)
                    n1438 = Equal To 0?(x=w1852) -> (x = 0?=w1853:bool)
                    n1439 = case shown="False" w1853 {
                      tunnel: w1852 -> [w1855 _]
                      tunnel: w1851 -> [w1854 _]
                      frame False {
                        w1857 = TRUE ("TRUE=HORA\nFALSE=GRAU")
                        # "AH tem sentido\ncontrário de RA"
                        n1440 = Divide(x=w1855, y=w1854) -> (x/y=w1856:dbl)
                        n1441 = call "Conversao Ms to Hora texto.vi"("TRUE=HORA\nFALSE=GRAU"=w1857, "PrecDEC"=w1856) -> ("Hora/Graus Texto Decimal"=w1858:string)
                        n1442 = call "Tx handeset.vi"("CMD On"="goRA", "Set Point"=w1858, "Estado do Botão"=w1857) -> ()  [unwired: 13 in]
                      }
                      frame True {
                      }
                    }
                  }
                }
              }
              event "BtPrecGO": Value Change {
                # "PROCESSO OFFSET"
                n1443 = event-data() -> ("NewVal"=w1862:bool)  [unwired: 1 in, 5 out]
                n1444 = property on="Delete Calagem" class="Bool"("Disabled"=u8 2) -> ()  [unwired: 2 in, 2 out]
                n1445 = case shown="True" w1862 {
                  tunnel: w1860 -> [_ w1863]
                  frame False {
                  }
                  frame True {
                    # "PROCESSO MOVE TELESCÓPIO"
                    n1446 = stacked-sequence {
                      tunnel: w1863 -> [_ w1871]
                      frame #0 {
                        n1447 = Not Equal To 0?(x="PreciseOffsetDEC") -> (x != 0?=w1865:bool)
                        n1448 = case shown="True" w1865 {
                          tunnel: "PreciseOffsetDEC" -> [_ w1866]
                          frame False {
                          }
                          frame True {
                            n1449 = call "Conversao Ms to Hora texto.vi"("TRUE=HORA\nFALSE=GRAU"=FALSE ("TRUE=HORA\nFALSE=GRAU"), "PrecDEC"=w1866) -> ("Hora/Graus Texto Decimal"=w1868:string)
                            n1450 = call "Tx handeset.vi"("CMD On"="goDEC", "Set Point"=w1868, "Estado do Botão"=TRUE ("TRUE=HORA\nFALSE=GRAU")) -> ()  [unwired: 13 in]
                          }
                        }
                      }
                      frame #1 {
                        n1451 = Not Equal To 0?(x="PreciseOffsetRA") -> (x != 0?=w1874:bool)
                        n1452 = Negate(x="PreciseOffsetRA") -> (-x=w1873:dbl)
                        n1453 = case shown="True" w1874 {
                          tunnel: w1873 -> [_ w1876]
                          tunnel: w1871 -> [_ w1875]
                          frame False {
                          }
                          frame True {
                            n1454 = Divide(x=w1876, y=w1875) -> (x/y=w1877:dbl)
                            n1455 = call "Conversao Ms to Hora texto.vi"("TRUE=HORA\nFALSE=GRAU"=TRUE ("TRUE=HORA\nFALSE=GRAU"), "PrecDEC"=w1877) -> ("Hora/Graus Texto Decimal"=w1879:string)
                            n1456 = call "Tx handeset.vi"("CMD On"="goRA", "Set Point"=w1879, "Estado do Botão"=TRUE ("TRUE=HORA\nFALSE=GRAU")) -> ()  [unwired: 13 in]
                          }
                        }
                      }
                    }
                  }
                }
              }
              event "Delete Calagem": Value Change {
                n1457 = event-data() -> ()  [unwired: 1 in, 6 out]
                n1458 = case shown="True" w1882 {
                  tunnel: 0.0 ("Calagem DEC Rel") -> [w1884 w1885]
                  frame False {
                    # "Local"
                    n1459 = global write "Global_Telescopio.vi" "CalAH Local"(w1884) -> ()
                    n1460 = global write "Global_Telescopio.vi" "CalDEC Local"(w1884) -> ()
                  }
                  frame True {
                    # "Global"
                    n1461 = global write "Global_Telescopio.vi" "Calagem AH"(w1885) -> ()
                    n1462 = global write "Global_Telescopio.vi" "Calagem DEC"(w1885) -> ()
                  }
                }
              }
              event "Calagem": Value Change {
                # "PROCESSO CALAGEM"
                n1463 = event-data() -> ()  [unwired: 1 in, 6 out]
                n1464 = global read "Global_Telescopio.vi" "CoordDia"() -> (w1887:bool)
                n1465 = global read "Global_Telescopio.vi" "CalGlobal"() -> (w1889:bool)
                n1466 = global read "Global_Telescopio.vi" "CalLocal"() -> (w1890:bool)
                n1467 = local read "ChkModel"() -> (w1891:bool)
                n1468 = local read "MeanRA"() -> (w1892:string)
                n1469 = local read "MeanDEC"() -> (w1888:string)
                n1470 = local read "PM_RA"() -> (w1893:string)
                n1471 = local read "PM_DEC"() -> (w1894:string)
                n1472 = local read "Temp amb"() -> (w1895:string)
                n1473 = local read "pressão atm"() -> (w1896:string)
                n1474 = local read "hum local"() -> (w1897:string)
                n1475 = call "PrecessaoCorrigida.vi"("Coordenada do dia"=w1887, "HabCorrModelo"=w1891, "UseLocalZero"=w1890, "UseGlobalZero"=w1889, "RA"=w1892, "DEC"=w1888, "MovProprioRA"=w1893, "MovProprioDEC"=w1894, "Temp amb (K)"=w1895, "Press atm (mB)"=w1896, "Humid relat"=w1897) -> ("RA"=w1899:dbl, "DEC"=w1898:dbl, "AH"=w1886:dbl)  [unwired: 2 out]
                n1476 = case shown="False" w1902 {
                  tunnel: w1899 -> [w1912 w1915]
                  tunnel: w1898 -> [w1904 w1917]
                  tunnel: w1901 -> [w1911 w1918]
                  tunnel: w1900 -> [w1913 w1916]
                  tunnel: w1886 -> [w1903 _]
                  frame False {
                    # "Local"
                    n1477 = Subtract(x=w1913, y=w1912) -> (x-y=w1914:dbl)
                    n1478 = Subtract(x=w1911, y=w1904) -> (x-y=w1908:dbl)
                    n1479 = global read "Global_Telescopio.vi" "CalAH Local"() -> (w1907:dbl)
                    n1480 = global read "Global_Telescopio.vi" "CalDEC Local"() -> (w1909:dbl)
                    n1481 = global write "Global_Telescopio.vi" "AH Zero Local"(w1903) -> ()
                    n1482 = global write "Global_Telescopio.vi" "DEC Zero Local"(w1904) -> ()
                    n1483 = Negate(x=w1914) -> (-x=w1910:dbl)
                    n1484 = Add(x=w1910, y=w1907) -> (x+y=w1906:dbl)
                    n1485 = Add(x=w1908, y=w1909) -> (x+y=w1905:dbl)
                    n1486 = global write "Global_Telescopio.vi" "CalAH Local"(w1906) -> ()
                    n1487 = global write "Global_Telescopio.vi" "CalDEC Local"(w1905) -> ()
                  }
                  frame True {
                    # "Global"
                    n1488 = stacked-sequence {
                      tunnel: w1918 -> [w1928 _ _]
                      tunnel: w1917 -> [w1927 _ _]
                      tunnel: w1916 -> [w1923 _ _]
                      tunnel: w1915 -> [w1922 _ _]
                      frame #0 {
                        w1919 = 0.0 ("CalAH Local")
                        n1489 = Subtract(x=w1923, y=w1922) -> (x-y=w1921:dbl)
                        n1490 = Subtract(x=w1928, y=w1927) -> (x-y=w1929:dbl)
                        n1491 = global read "Global_Telescopio.vi" "Calagem AH"() -> (w1926:dbl)
                        n1492 = global read "Global_Telescopio.vi" "Calagem DEC"() -> (w1931:dbl)
                        n1493 = Negate(x=w1921) -> (-x=w1924:dbl)
                        n1494 = local write "Processa Centragem"(TRUE) -> ()
                        n1495 = Add(x=w1924, y=w1926) -> (x+y=w1925:dbl)
                        n1496 = Add(x=w1929, y=w1931) -> (x+y=w1930:dbl)
                        n1497 = global write "Global_Telescopio.vi" "Calagem AH"(w1925) -> ()
                        n1498 = global write "Global_Telescopio.vi" "CalAH Local"(w1919) -> ()
                        n1499 = global write "Global_Telescopio.vi" "CalDEC Local"(w1919) -> ()
                        n1500 = global write "Global_Telescopio.vi" "Calagem DEC"(w1930) -> ()
                      }
                      frame #1 {
                        # "25/10/2012 - Sempre que o usuario faz uma \ncalagem global, o valor da calagem e'  salva \nautomaticamente em GLOBAIS_CALAGEM.DAT"
                        n1501 = call "Salva_Calagem_Global.vi"() -> ()  [unwired: 1 in]
                      }
                      frame #2 {
                        # "Salva no Logo valor \ndo deslocamento da \ncalagem global"
                        n1502 = local read "DeslocDEC"() -> (w1932:dbl)
                        n1503 = local read "DeslocRA"() -> (w1933:dbl)
                        n1504 = call "Log_Calagem.vi"("Desloc DEC"=w1932, "Desloc RA"=w1933, "File Name"="LOG_COMANDOS.TXT") -> ()  [unwired: 3 in]
                      }
                    }
                  }
                }
              }
              event "Up HS": Value Change {
                w1937 = u8 0 ("Disabled")
                n1505 = event-data() -> ("NewVal"=w1936:bool)  [unwired: 1 in, 5 out]
                n1506 = call "Tx handeset.vi"("CMD On"="up" ("Comando"), "CMD Off"="stopv" ("Comando"), "Estado do Botão"=w1936, "Velocity (arcsec/sec)"=w1940) -> ()  [unwired: 12 in]
                n1507 = local write "MOV_IDX_DEC"(w1936) -> ()
                n1508 = property on="Delete Calagem" class="Bool"("Disabled"=w1937) -> ()  [unwired: 2 in, 2 out]
                n1509 = Select(t=u8 2 ("Disabled"), s=FALSE, f=w1937) -> (s? t:f=w1938:u8)
                n1510 = property on="Down HS" class="Bool (strict)"("Disabled"=w1938) -> ()  [unwired: 2 in, 2 out]
              }
            }
            n1511 = Subtract(x=w1792, y=w1804) -> (x-y=w1801:dbl)
            n1512 = Subtract(x=w1794, y=w1803) -> (x-y=w1805:dbl)
            n1513 = Multiply(x=w1801, y=w1798) -> (x*y=w1802:dbl)
            n1514 = global read "Global_Telescopio.vi" "ObjCentrado"() -> (w1795:bool)
            n1515 = call "Rad to Arcsec.vi"("Radiano"=w1802) -> ("Arcsec"=w1788:dbl)
            n1516 = call "Rad to Arcsec.vi"("Radiano"=w1805) -> ("Arcsec"=w1787:dbl)
            n1517 = case shown="False" w1795 {
